vi "Overflowvi.vi"(10 "limit":dbl=1.0 format="%#_13g", 11 "value":dbl format="%#_13g") -> (3 "overflow":dbl)   [LabVIEW 2019, in "DriveOld.lvlib" / "Drive.lvclass"]
doc: "For a given value, and a given limit, this vi gives you the amount of the value that exceeds the limit. It preserves sign, so positive indicates greater than the limit, negative indicates less than the limit. Limits are symmetrical about zero."
uses:
  Drive.lvclass
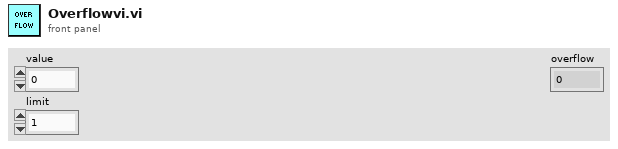
[diagram p1: front panel]
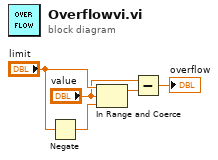
[diagram p0: block diagram]
diagram:
  n1 = Negate(x="limit") -> (-x=w5:dbl)
  n2 = In Range and Coerce(upper limit="limit", x="value", lower limit=w5) -> (coerced(x)=w3:dbl)  [unwired: 1 out]
  n3 = Subtract(x="value", y=w3) -> (x-y=→"overflow":dbl)
